vi "User (multiple).vi"(7 "User.lvclass":refnum<class "User.lvclass">, 8 "error in (no error)":errorcluster, 11 "XY-data":cluster{"X-array":dbl[], "Y-array":dbl[]}[](array[cluster]) {"Y-array" format="%.2p"; "X-array" format="%.2p"}) -> (0 "error out":errorcluster, 3 "XY-data out":cluster{"X-array":dbl[], "Y-array":dbl[]}[](array[cluster]) {"Y-array" format="%.2p"; "X-array" format="%.2p"}, 5 "User.lvclass out":refnum<class "User.lvclass">)   [LabVIEW 2019, in "User.lvclass"]
doc: "Call user code by selecting an override with <b>User.lvclass</b>."
uses:
  User.lvclass
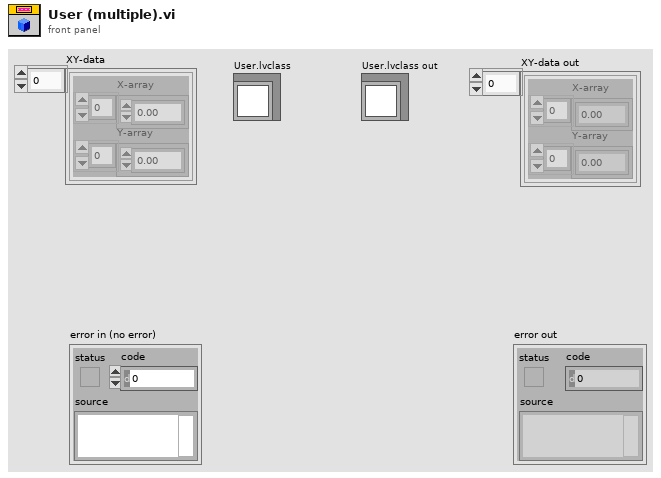
[diagram p1: front panel]
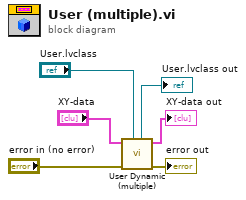
[diagram p0: block diagram]
diagram:
  n1 = call-dynamic "User Dynamic (multiple).vi"("User.lvclass"="User.lvclass", "error in (no error)"="error in (no error)", "XY-data"="XY-data") -> ("error out"=→"error out":errorcluster, "XY-data out"=→"XY-data out":cluster{"X-array":dbl[], "Y-array":dbl[]}[], "User.lvclass out"=→"User.lvclass out":refnum<class "User.lvclass">)  [unwired: 6 in]
